vi "WriteWebView.vi"(8 "Error In":errorcluster, 10 "WebView":refnum<class "WebView2 Control.lvclass">, 11 "object in":refnum<class "Component.lvclass">) -> (0 "Error Out":errorcluster, 3 "object out":refnum<class "Component.lvclass">)   [LabVIEW 2020, in "Component.lvclass"]
uses:
  Component.lvclass
  <vilib>/sklein/WebView2/Webview2 Lib/WebView2 Control Object/WebView2 Control.lvclass
  Component.lvclass/Component.ctl
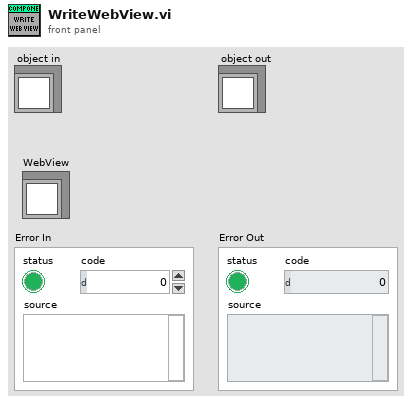
[diagram p1: front panel]
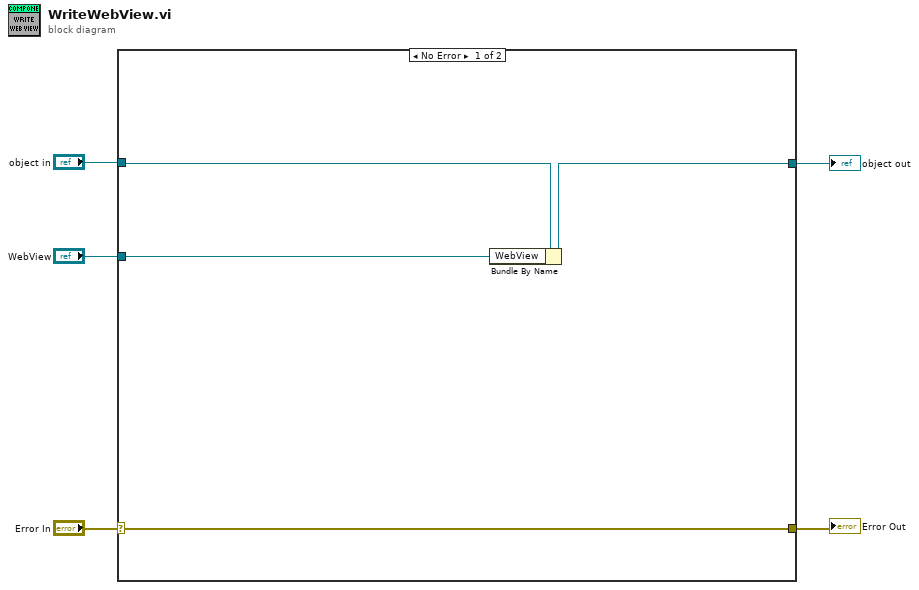
[diagram p0: block diagram]
diagram:
  n1 = case shown="No Error" "Error In" {
    selector: "Error In" -> [w8 w11]
    tunnel: [w8 w11] -> w4
    tunnel: [w6 w10] -> w2
    tunnel: "object in" -> [w7 w10]
    tunnel: "WebView" -> [w9 _]
    frame No Error {
      n2 = Bundle By Name(cluster=w7, "WebView"=w9) -> (w6:refnum<class "Component.lvclass">)
    }
    frame Error {
    }
  }
  "Error Out" <- w4
  "object out" <- w2
